vi "Plugin Inline Rx.vi"(8 "error in (no error)":errorcluster, 9 "framework iteration":u64, 10 "Dispatcher Interface in":refnum<class "Dispatcher Interface.lvclass">, 11 "Plugin Schedule in":T1) -> (0 "error out":errorcluster, 2 "Dispatcher Interface out":refnum<class "Dispatcher Interface.lvclass">, 3 "Plugin Schedule out":T1)   [LabVIEW 2017, in "DSF Core.lvlib" / "Scheduler.lvclass"]
uses:
  Scheduler.lvclass
  Timing/Timing.lvclass
  Interfaces/Dispatcher/Dispatcher Interface.lvclass
  Timing/Plugin Timing Group.lvclass
  C:/Git/DSF/Data Sharing Framework/Source/Core/Engine/Classes/Timing/Timing.lvclass
  Plugin Scheduler Data.ctl
  Timing/Transfer Group Timing.lvclass
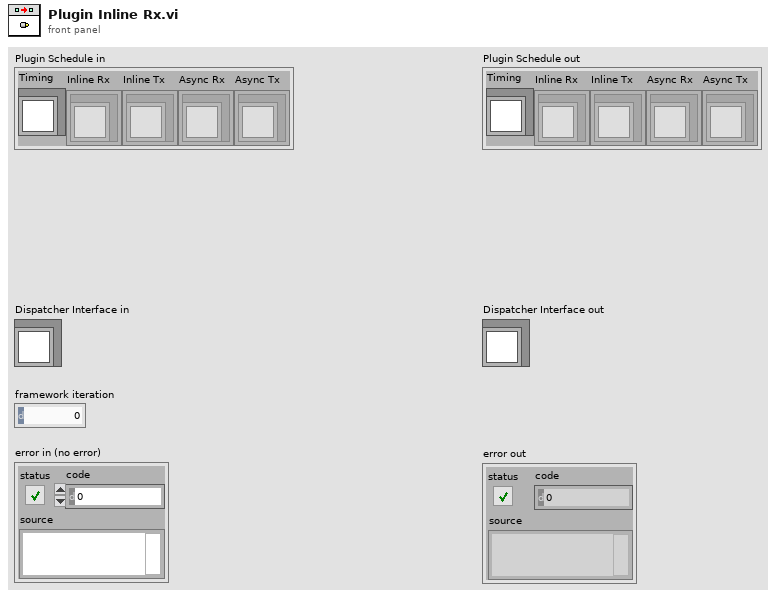
[diagram p1: front panel]
types:
  T1 = typedef "DSF Core.lvlib/Scheduler.lvclass/Plugin Scheduler Data.ctl" = cluster{"Timing":refnum<class "Plugin Timing Group.lvclass">, "Inline Rx":refnum<class "Transfer Group Timing.lvclass">[], "Inline Tx":refnum<class "Transfer Group Timing.lvclass">[], "Async Rx":refnum<class "Transfer Group Timing.lvclass">[], "Async Tx":refnum<class "Transfer Group Timing.lvclass">[]}
  T2 = typedef "DSF Core.lvlib/Scheduler.lvclass/Transfer Group Scheduler Data.ctl" = cluster{"Timing":refnum<class "Timing.lvclass">, "ID":i32, "Return FIFO":refnum<k33>}
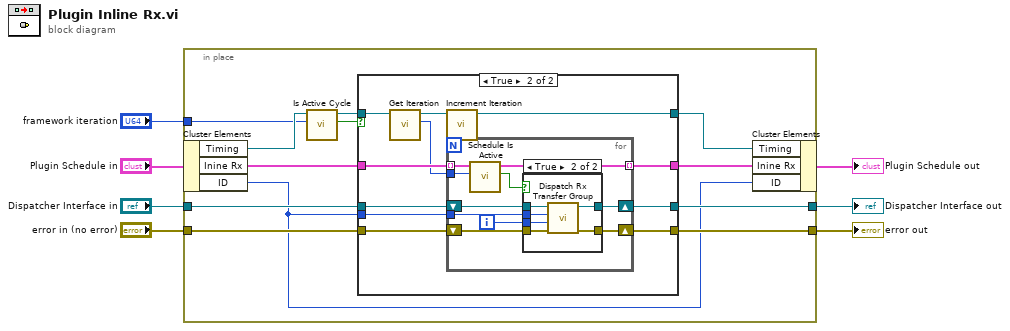
[diagram p0: block diagram]
diagram:
  n1 = in-place {
    in-place-border: "framework iteration" -> [w13]
    in-place-border: "Dispatcher Interface in" -> [w12]
    in-place-border: [w11] -> w4
    in-place-border: [w10] -> w2
    in-place-border: "error in (no error)" -> [w9]
    n2 = in-place-cluster #1("Plugin Schedule in") -> ("Timing"=w15:refnum<class "Plugin Timing Group.lvclass">, "Inine Rx"=w19:T2[], "ID"=w8:i32)
    n3 = call "Is Active Cycle.vi"("iteration"=w13, "Timing in"=w15) -> ("active?"=w17:bool, "Timing out"=w16:refnum<class "Plugin Timing Group.lvclass">)  [unwired: 8 in]
    n4 = case shown="True" w17 {
      tunnel: w19 -> [w23 w34]
      tunnel: [w23 w33] -> w18
      tunnel: w16 -> [w22 w32]
      tunnel: [w22 w24] -> w14
      tunnel: w12 -> [w21 w29]
      tunnel: [w21 w28] -> w11
      tunnel: [w20 w27] -> w10
      tunnel: w8 -> [_ w26]
      tunnel: w9 -> [w20 w25]
      frame False {
      }
      frame True {
        n5 = call "Get Iteration.vi"("Timing in"=w32) -> ("Iteration"=w31:u64, "Timing out"=w30:refnum<class "Plugin Timing Group.lvclass">)  [unwired: 9 in]
        n6 = call "Increment Iteration.vi"("Timing in"=w30) -> ("Timing out"=w24:refnum<class "Plugin Timing Group.lvclass">)  [unwired: 10 in]
        n7 = for {
          tunnel: w34 -> [w44] mode=indexing
          tunnel: [w43] -> w33 mode=indexing
          tunnel: w31 -> [w42]
          shift-right: [w40] -> w28
          shift-left: w29 -> [w41]
          shift-right: [w39] -> w27
          shift-left: w25 -> [w38]
          tunnel: w26 -> [w37]
          i -> [w36]
          n8 = call "Schedule Is Active.vi"("iteration"=w42, "Schedule in"=w44) -> ("active?"=w35:bool, "Schedules out"=w43:T2)  [unwired: 8 in]
          n9 = case shown="True" w35 {
            tunnel: w41 -> [w46 w52]
            tunnel: [w46 w51] -> w40
            tunnel: [w45 w50] -> w39
            tunnel: w38 -> [w45 w49]
            tunnel: w37 -> [_ w48]
            tunnel: w36 -> [_ w47]
            frame False {
            }
            frame True {
              n10 = call "Dispatch Rx Transfer Group.vi"("error in (no error)"=w49, "Transfer Group ID"=w47, "Plugin ID"=w48, "Dispatcher Interface in"=w52) -> ("error out"=w50:errorcluster, "Dispatcher Interface out"=w51:refnum<class "Dispatcher Interface.lvclass">)  [unwired: 6 in]
            }
          }
        }
      }
    }
    n11 = in-place-cluster #1("Timing"=w14, "Inine Rx"=w18, "ID"=w8) -> (→"Plugin Schedule out":T1)
  }
  "Dispatcher Interface out" <- w4
  "error out" <- w2
